vi "Get Target List.vi"(8 "error in (no error)":errorcluster, 11 "SysDef Refnum in":refnum<k24>) -> (0 "error out":errorcluster, 2 "Target List Refnums":refnum<k24>[](array[refnum]), 3 "SysDef Refnum out":refnum<k24>)   [LabVIEW 2019, in "Scalar Channels Testing.lvclass"]
uses:
  Scalar Channels Testing.lvclass
  NationalInstruments.VeriStand.SystemDefinitionAPI
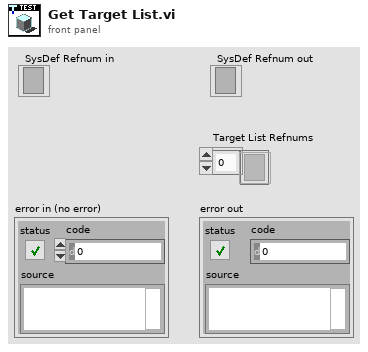
[diagram p1: front panel]
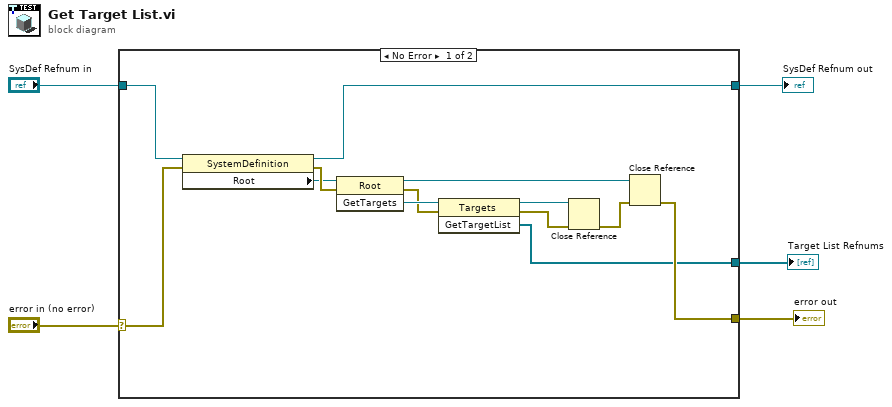
[diagram p0: block diagram]
diagram:
  n1 = case shown="No Error" "error in (no error)" {
    selector: "error in (no error)" -> [w6 w19]
    tunnel: "SysDef Refnum in" -> [w11 w20]
    tunnel: [w9 w19] -> w4
    tunnel: [w8 _] -> w3
    tunnel: [w7 w20] -> w2
    frame No Error {
      n2 = property class="SystemDefinition"(reference=w11, error in=w6) -> (reference out=w7:refnum<k24>, error out=w13:errorcluster, "Root"=w12:refnum<k24>)
      n3 = invoke class="Root" method="GetTargets"(reference=w12, error in=w13) -> (reference out=w16:refnum<k24>, error out=w10:errorcluster, "GetTargets"=w14:refnum<k24>)  [unwired: 1 in]
      n4 = invoke class="Targets" method="GetTargetList"(reference=w14, error in=w10) -> (reference out=w17:refnum<k24>, error out=w18:errorcluster, "GetTargetList"=w8:refnum<k24>[])  [unwired: 1 in]
      n5 = Close Reference(reference=w17, error in (no error)=w18) -> (error out=w15:errorcluster)
      n6 = Close Reference(reference=w16, error in (no error)=w15) -> (error out=w9:errorcluster)
    }
    frame Error {
    }
  }
  "error out" <- w4
  "Target List Refnums" <- w3
  "SysDef Refnum out" <- w2
